vi "init.vi"(8 "error in (no error)":errorcluster, 11 "ForceSensor in":refnum<class "ForceSensorCalculator_Axial.lvclass">) -> (0 "error out":errorcluster, 3 "ForceSensor out":refnum<class "ForceSensorCalculator_Axial.lvclass">)   [LabVIEW 2015, in "ForceSensorCalculator_Axial.lvclass"]
uses:
  ForceSensorCalculator_Axial.lvclass
  <userlib>/Common/Devices/ForceSensorCalculator/Config/ForceSensorCalculator.ctl
  <userlib>/Common/Devices/ForceSensorCalculator/ForceSensorCalculator/ForceSensorCalculator.lvclass/ForceSensorCalculator.ctl
  <userlib>/Common/Devices/ForceSensorCalculator/ForceSensorCalculator/ForceSensorCalculator.lvclass
  <userlib>/Common/Devices/ForceSensorCalculator/ForceSensorCalculator.lvlib
  ConfigurationThisComponent/ConfigurationThisComponent.lvclass
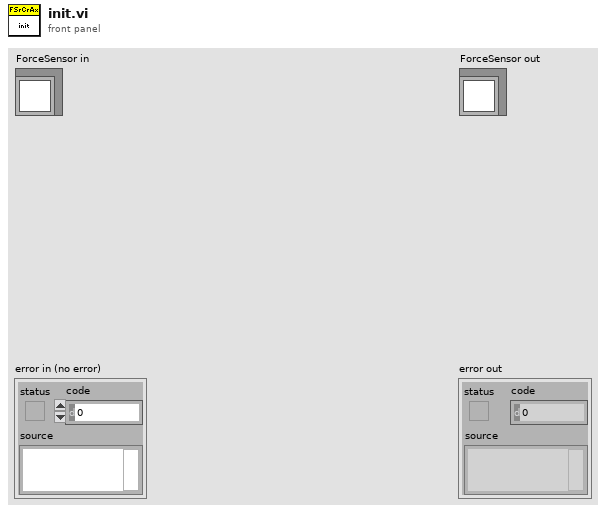
[diagram p1: front panel]
types:
  T1 = typedef "ForceSensorCalculator.lvlib/ForceSensorCalculator.ctl" = cluster{"Capacity":dbl[unit], "Sensitivity":dbl[unit]}
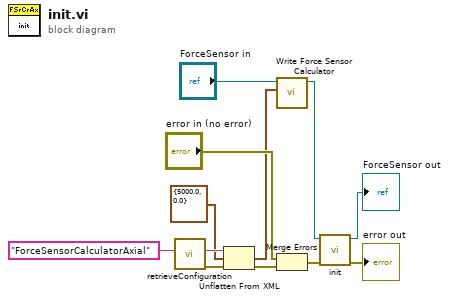
[diagram p0: block diagram]
diagram:
  n1 = call "retrieveConfiguration.vi"("configName"="ForceSensorCalculatorAxial") -> ("error out"=w9:errorcluster, "xmlConfig"=w8:string)  [unwired: 8 in, 1 out]
  n2 = Unflatten From XML(xml string=w8, type=T1 {"Capacity"=5000.0, "Sensitivity"=0.0} ("Force Sensor"), error in (no error)=w9) -> (value=w1:T1, error out=w5:errorcluster)
  n3 = call <userlib>:"Write Force Sensor Calculator.vi"("Force Sensor Calculator"=w1, "ForceSensorCalculator in"="ForceSensor in") -> ("ForceSensorCalculator out"=w2:refnum<class "ForceSensorCalculator_Axial.lvclass">)  [unwired: 9 in]
  n4 = Merge Errors("error in (no error)", w5) -> (w4:errorcluster)
  n5 = call-parent "init.vi"("error in (no error)"=w4, "ForceSensor in"=w2) -> ("error out"=→"error out":errorcluster, "ForceSensor out"=→"ForceSensor out":refnum<class "ForceSensorCalculator_Axial.lvclass">)  [unwired: 8 in]
